vi "Auth Method.vi"(11 "IAuthenticator in":refnum<class "IAuthenticator.lvclass">) -> (2 "Authmethod":string, 3 "IAuthenticator out":refnum<class "IAuthenticator.lvclass">)   [LabVIEW 2020, in "wamplv.lvlib" / "IAuthenticator.lvclass"]
uses:
  IAuthenticator.lvclass
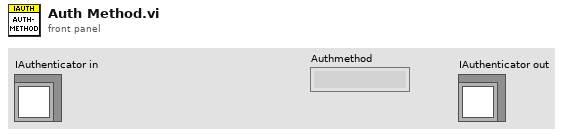
[diagram p1: front panel]
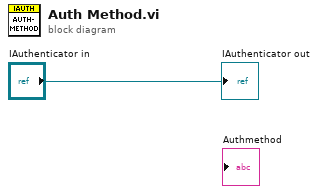
[diagram p0: block diagram]
diagram:
  "IAuthenticator out" <- "IAuthenticator in"
